vi "What.vi"(5 "Average During Loop ?":bool, 6 "# of Loops":u32, 7 "Action 2":T1 caption="Action", 8 "Program":T2(array[cluster]), 9 "Loop ?":cluster{i32, i32}, 10 "reference":refnum<vi>) -> (0 "Preview":cluster{dbl[], dbl[]}[](array[cluster]), 1 "Array 3":dbl[](array[numeric]), 2 "Array":bool[](array[boolean]), 3 "Array 2":bool[](array[boolean]), 4 "Action":T1)   [LabVIEW 2018]
uses:
  Multi Segment Waveform.xctl
  <vilib>/_xctls/Action.ctl
  <vilib>/_xctls/XControlSupport.lvlib
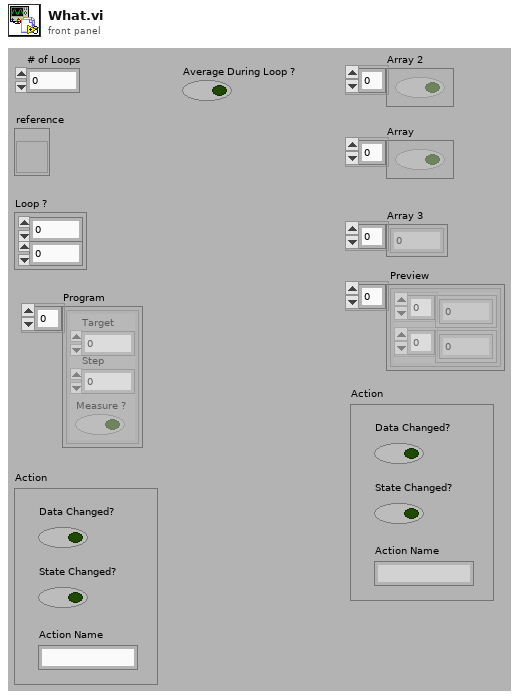
[diagram p1: front panel]
types:
  T1 = typedef "XControlSupport.lvlib/Action.ctl" = cluster{"Data Changed?":bool, "State Changed?":bool, "Action Name":string}
  T2 = cluster{"Target":dbl, "Step":dbl, "Measure ?":bool}[]
  T3 = cluster{"Target":dbl, "Step":dbl, "Measure ?":bool}
  T4 = cluster{"Storage Locs":i32[], "Measure":bool[], "Field":dbl[], "Direction":bool[]}
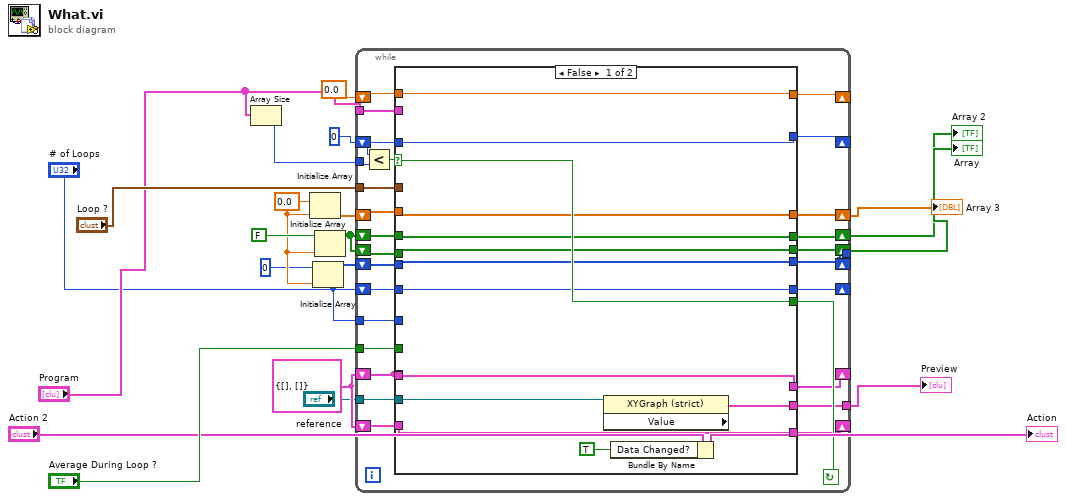
[diagram p0: block diagram]
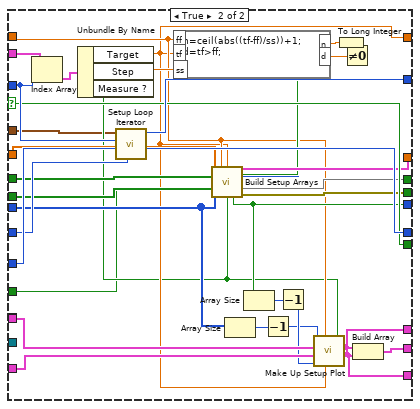
[diagram p2: hidden frame]
diagram:
  w10 = cluster{dbl[], dbl[]} {[], []}
  w7 = 0.0
  n1 = Array Size(array="Program") -> (size(s)=w14:i32)
  n2 = Initialize Array(w7, w7) -> (w12:dbl[])
  n3 = Initialize Array(0, w7) -> (w8:i32[])
  n4 = Initialize Array(FALSE, w7) -> (w5:bool[])
  n5 = while {
    shift-left: w5 -> [w28]
    shift-right: [w27] -> w19
    tunnel: [w29] -> _
    shift-left: w8 -> [w30]
    shift-right: [w29] -> _
    tunnel: "# of Loops" -> [w31]
    shift-left: w10 -> [w35]
    shift-right: [w34] -> _
    shift-left: w10 -> [w32]
    shift-right: [w33] -> _
    shift-left: w12 -> [w39]
    shift-right: [w38] -> w17
    shift-left: "# of Loops" -> [w44]
    shift-right: [w43] -> _
    tunnel: w14 -> [w47]
    shift-left: 0 -> [w49]
    shift-right: [w42] -> _
    shift-left: w5 -> [w37]
    shift-right: [w36] -> w18
    shift-left: 0.0 -> [w41]
    shift-right: [w40] -> _
    tunnel: "Program" -> [w48]
    tunnel: "Loop ?" -> [w26]
    tunnel: [w25] -> w22
    tunnel: "Average During Loop ?" -> [w24]
    tunnel: "reference" -> [w23]
    stop <- w45 continue-if-true
    n6 = Less?(x=w49, y=w47) -> (x < y?=w46:bool)
    n7 = case shown="False" w46 {
      selector: w46 -> [w61 w84]
      tunnel: w49 -> [w59 w89]
      tunnel: w48 -> [_ w96]
      tunnel: [w61 w84] -> w45
      tunnel: w44 -> [w60 w87]
      tunnel: [w60 w86] -> w43
      tunnel: [w59 w85] -> w42
      tunnel: w41 -> [w58 w67]
      tunnel: [w58 w66] -> w40
      tunnel: w39 -> [w57 w83]
      tunnel: [w57 w80] -> w38
      tunnel: w37 -> [w56 w82]
      tunnel: [w56 w81] -> w36
      tunnel: w32 -> [_ w92]
      tunnel: w35 -> [w54 w91]
      tunnel: [w54 w94] -> w34
      tunnel: [w55 w93] -> w33
      tunnel: w32 -> [w55 _]
      tunnel: w31 -> [_ w88]
      tunnel: w30 -> [w53 w69]
      tunnel: [w53 w73] -> w29
      tunnel: w28 -> [w52 w75]
      tunnel: [w52 w74] -> w27
      tunnel: w26 -> [_ w64]
      tunnel: [w51 w63] -> w25
      tunnel: w24 -> [_ w62]
      tunnel: w23 -> [w50 _]
      frame False {
        n8 = property class="XYGraph (strict)"(reference=w50) -> ("Value"=w51:cluster{dbl[], dbl[]}[])  [unwired: 1 in, 2 out]
      }
      frame True {
        n9 = Index Array(array=w96, index=w89) -> (element=w95:T3)
        n10 = Unbundle By Name(w95) -> ("Target"=w66:dbl, "Step"=w90:dbl, "Measure ?"=w65:bool)
        n11 = call "Setup Loop Iterator.vi"("Loop Iterator"=w87, "Total Loops"=w88, "Previous Line"=w89, "Loop"=w64) -> ("Loop Iterator Out"=w86:u32, "Line Iterator Out"=w85:i32)  [unwired: 4 out]
        n12 = formula code="n=ceil(abs((tf-ff)/ss))+1;\nd=tf>ff;"("ff"=w67, "tf"=w66, "ss"=w90) -> ("n"=w77:dbl, "d"=w79:dbl)
        n13 = Array Size(array=w69) -> (size(s)=w70:i32)
        n14 = Decrement(x=w70) -> (x-1=w68:i32)
        n15 = To Long Integer(number=w77) -> (32bit integer=w76:i32)
        n16 = Not Equal To 0?(x=w79) -> (x != 0?=w78:bool)
        n17 = call "Build Setup Arrays.vi"("Preview In"=w83, "Measure ?"=w67, "First Field"=w66, "N Points"=w78, 5:w82, 6:w76, 9:w75, "error in (no error)"=w69, "Last Field"=w62, "Direction"=w65) -> ("Preview Out"=w80:T4, 10:w81, "Average During Loop ?"=w73:bool, "error out"=w74:errorcluster)  [unwired: 2 out]
        n18 = Array Size(array=w73) -> (size(s)=w72:i32)
        n19 = Decrement(x=w72) -> (x-1=w71:i32)
        n20 = call "Make Up Setup Plot.vi"("Put in plot 1"=w65, "End Field"=w66, "Start Field"=w67, "End X"=w71, "Plot 2 In"=w91, "Plot 1 In"=w92, "Start X"=w68) -> ("Plot 2 Out"=w94:cluster{dbl[], dbl[]}, "Plot 1 Out"=w93:cluster{dbl[], dbl[]})  [unwired: 1 in]
        n21 = Build Array(w93, w94) -> (w63:cluster{dbl[], dbl[]}[])
      }
    }
  }
  "Preview" <- w22
  "Array" <- w19
  "Array 2" <- w18
  "Array 3" <- w17
  n22 = Bundle By Name(cluster="Action 2", "Data Changed?"=TRUE) -> (→"Action":T1)
